vi "Spatial Dual Decode Packet 33 (SubVI).vi"(8 "SGL Precision":i16=6, 10 "Packet 33 Bytes In":u8[](array[numeric])) -> (0 "Channel Data Type":string[](array[string])=["Float", "Float", "Float"], 1 "Channel Units":string[](array[string])=["m/s/s", "m/s/s", "m/s/s"], 2 "Data":string[](array[string]), 3 "Channel Names":string[](array[string])=["Acc X", "Acc Y", "Acc Z"], 4 "Packet 33 Decoded Data Cluster":T1)   [LabVIEW 2019, in "SpatialDual_Parsers.lvlib"]
uses:
  SpatialDual_Parsers.lvlib
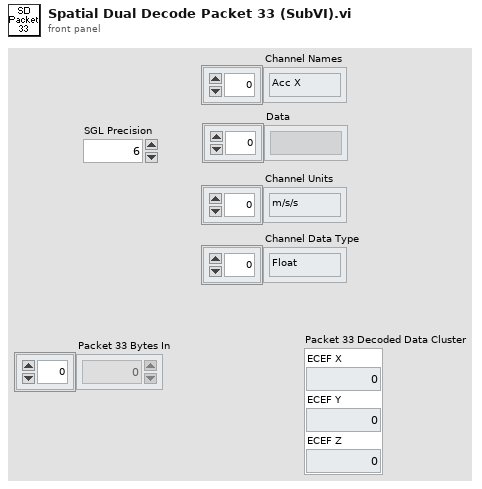
[diagram p1: front panel]
types:
  T1 = cluster{"ECEF X":dbl, "ECEF Y":dbl, "ECEF Z":dbl}
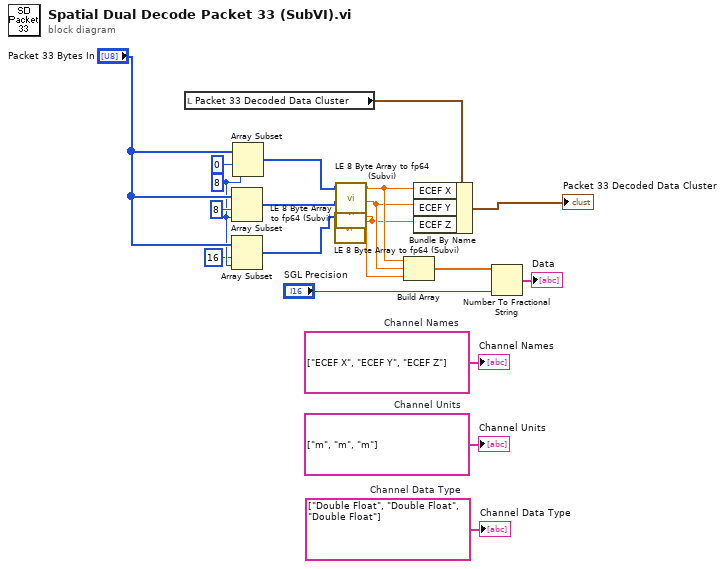
[diagram p0: block diagram]
diagram:
  w7 = string[] ["Double Float", "Double Float", "Double Float"]  # Channel Data Type
  w8 = string[] ["m", "m", "m"]  # Channel Units
  w9 = string[] ["ECEF X", "ECEF Y", "ECEF Z"]  # Channel Names
  w14 = 8 ("length")
  n1 = local read "Packet 33 Decoded Data Cluster"() -> (w19:T1)
  n2 = Array Subset(array="Packet 33 Bytes In", index=8, length=w14) -> (w5:u8[])
  n3 = Array Subset(array="Packet 33 Bytes In", index=16, length=w14) -> (w4:u8[])
  n4 = Array Subset(array="Packet 33 Bytes In", index=0, length=w14) -> (w6:u8[])
  n5 = call "LE 8 Byte Array to fp64 (Subvi).vi"("8 Bytes in"=w4) -> ("fp64 Out"=w1:dbl)  [unwired: 8 in]
  n6 = call "LE 8 Byte Array to fp64 (Subvi).vi"("8 Bytes in"=w6) -> ("fp64 Out"=w3:dbl)  [unwired: 8 in]
  n7 = call "LE 8 Byte Array to fp64 (Subvi).vi"("8 Bytes in"=w5) -> ("fp64 Out"=w2:dbl)  [unwired: 8 in]
  n8 = Build Array(w3, w2, w1) -> (w12:dbl[])
  n9 = Bundle By Name(cluster=w19, "ECEF X"=w3, "ECEF Y"=w2, "ECEF Z"=w1) -> (→"Packet 33 Decoded Data Cluster":T1)
  n10 = Number To Fractional String(number=w12, precision (6)="SGL Precision") -> (F-format string=→"Data":string[])  [unwired: 2 in]
  "Channel Names" <- w9
  "Channel Units" <- w8
  "Channel Data Type" <- w7
